vi "BinaryStringToValue (Array).vi"(1 "Array string":string[](array[string])) -> (0 "Array value":u8[](array[numeric]))   [LabVIEW 2011, in "UintClass.lvclass"]
uses:
  UintClass.lvclass
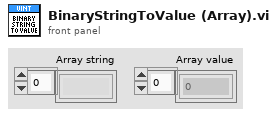
[diagram p1: front panel]
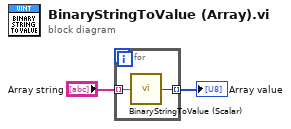
[diagram p0: block diagram]
diagram:
  n1 = for {
    tunnel: "Array string" -> [w4] mode=indexing
    tunnel: [w3] -> w1 mode=indexing
    n2 = call "BinaryStringToValue (Scalar).vi"("String"=w4) -> ("Value"=w3:u8)
  }
  "Array value" <- w1
